vi "Loadcell CYL Home.vi"(7 "Model Name":T1, 8 "Error In":errorcluster, 9 "Intialize?":bool=TRUE, 10 "Inputs":T2) -> (0 "error out":errorcluster, 1 "Completed":bool, 4 "Status":cluster{"Status":string, "Elapsed Time":dbl})   [LabVIEW 2017]
uses:
  controls/All Inputs.ctl
  controls/SACB DI.ctl
  controls/Model Name.ctl
  controls/Loadcell CYL Home.ctl
  controls/FGV DO.ctl
panel:
  in  "Delay (for De-Clamp)":u32=500
  in  "Timeout (ms)":u32=15000
  # "Inputs"
  # "Variables"
  # "Outputs"
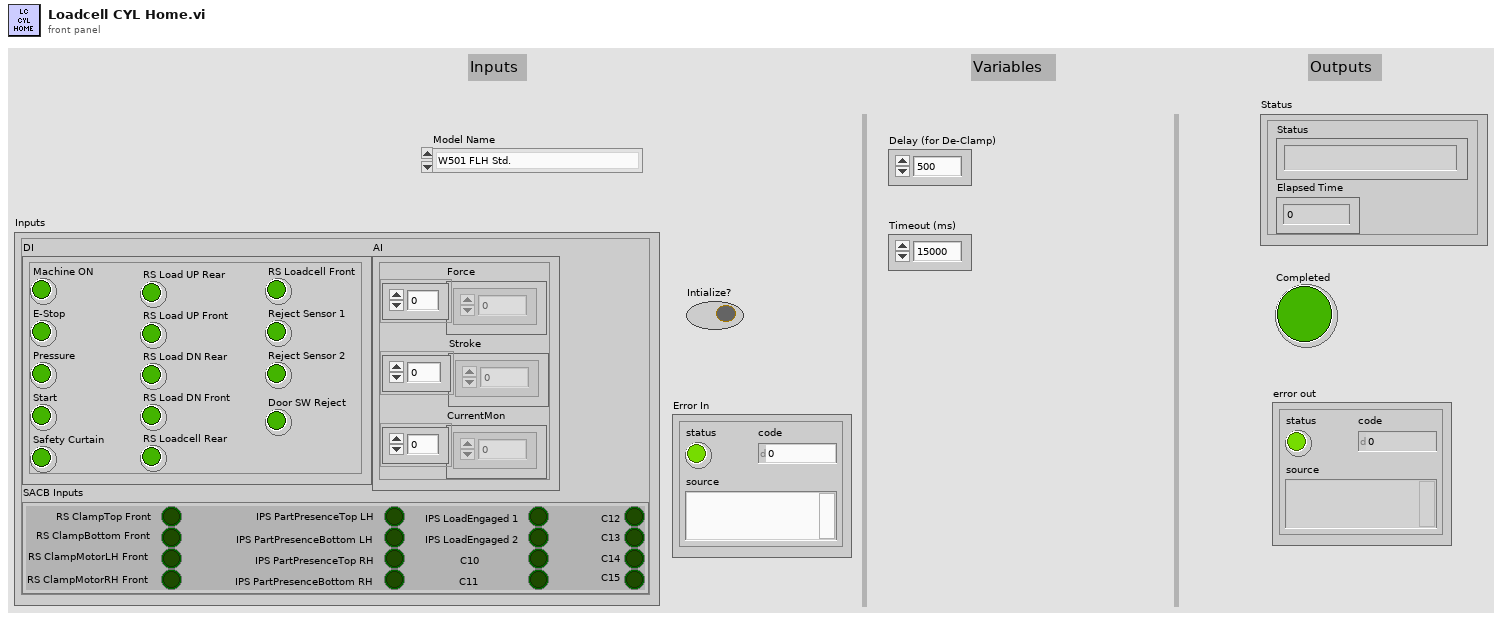
[diagram p1: front panel]
types:
  T1 = typedef "Model Name.ctl" = enum16{"W501 FLH Std.", "W501 FRH Std."}
  T2 = typedef "All Inputs.ctl" = cluster{"DI":cluster{"Machine ON":bool, "E-Stop":bool, "Pressure":bool, "Start":bool, "Safety Curtain":bool, "RS Load UP Rear":bool, "RS Load UP Front":bool, "RS Load DN Rear":bool, "RS Load DN Front":bool, "RS Loadcell Rear":bool, "RS Loadcell Front":bool, "Reject Sensor 1":bool, "Reject Sensor 2":bool, "Door SW Reject":bool}, "AI":cluster{"Force":dbl[], "Stroke":dbl[], "CurrentMon":dbl[]}, "SACB Inputs":T3}
  T3 = typedef "SACB DI.ctl" = cluster{"RS ClampTop Front":bool, "RS ClampBottom Front":bool, "RS ClampMotorLH Front":bool, "RS ClampMotorRH Front":bool, "IPS PartPresenceTop LH":bool, "IPS PartPresenceBottom LH":bool, "IPS PartPresenceTop RH":bool, "IPS PartPresenceBottom RH":bool, "IPS LoadEngaged 1":bool, "IPS LoadEngaged 2":bool, "C10":bool, "C11":bool, "C12":bool, "C13":bool, "C14":bool, "C15":bool}
  T4 = typedef "Loadcell CYL Home.ctl" = enum16{"Initialize", "Loadcell CYL to Home", "Delay", "Done", "Error"}
  T5 = typedef "FGV DO.ctl" = enum16{"Initialize", "Start Task", "Clamping", "Load CYL", "Contactors", "Loadcell CYL", "BSL", "Read DO", "Clear Tasks", "Clear Task"}
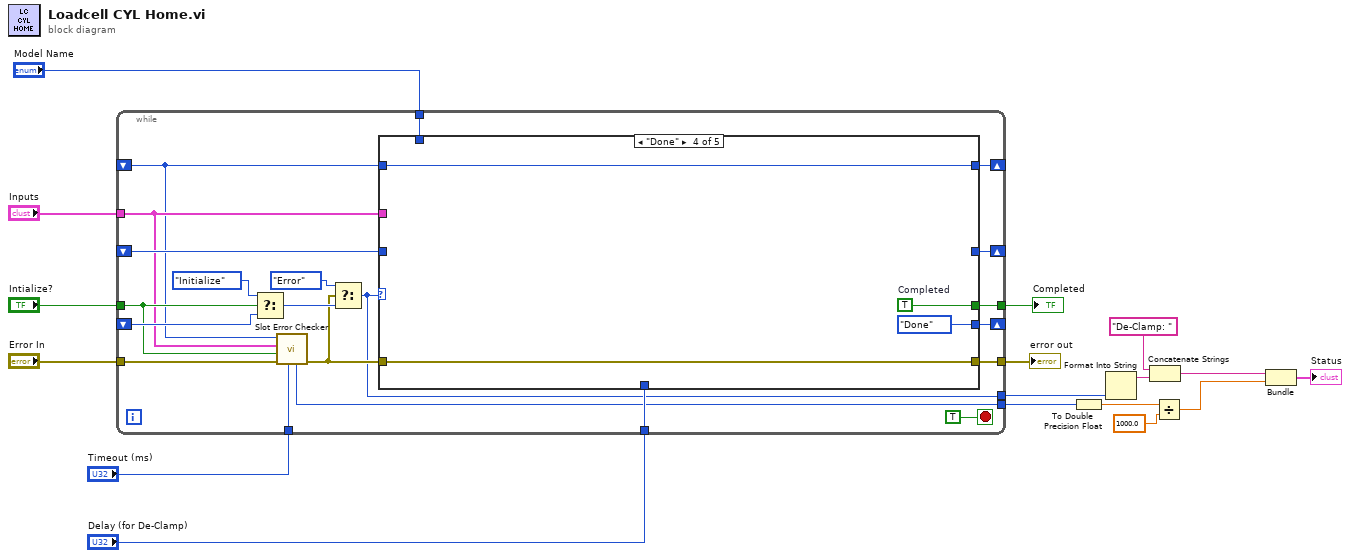
[diagram p0: block diagram]
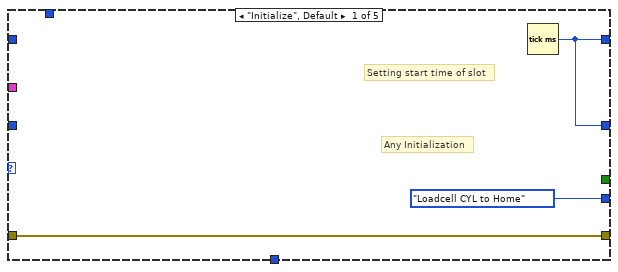
[diagram p2: hidden frame]
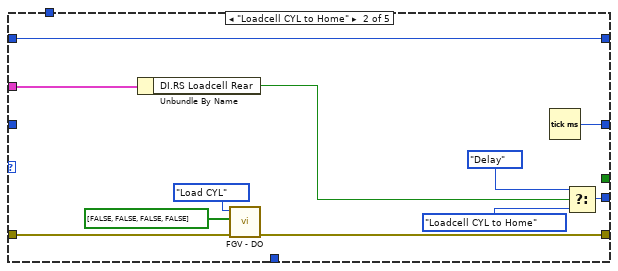
[diagram p3: hidden frame]
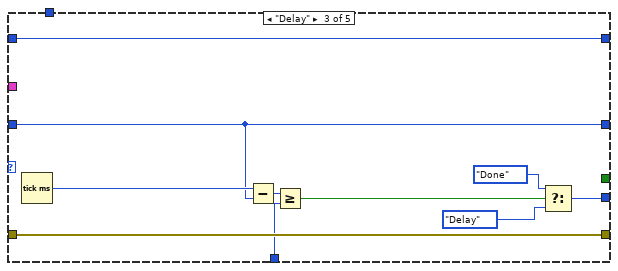
[diagram p4: hidden frame]
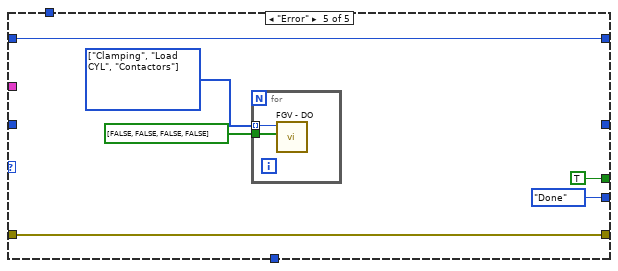
[diagram p5: hidden frame]
diagram:
  n1 = while {
    tunnel: "Intialize?" -> [w28]
    shift-right: [w35] -> _
    shift-left: _ -> [w37]
    shift-right: [w34] -> _
    shift-left: _ -> [w33]
    tunnel: "Error In" -> [w29]
    tunnel: [w32] -> w17
    tunnel: [w31] -> w16
    tunnel: "Inputs" -> [w27]
    shift-right: [w30] -> _
    shift-left: _ -> [w26]
    tunnel: "Delay (for De-Clamp)" -> [w22]
    tunnel: "Timeout (ms)" -> [w21]
    tunnel: [w20] -> w10
    tunnel: [w19] -> w7
    tunnel: "Model Name" -> [w18]
    stop <- TRUE stop-if-true
    n2 = Select(t=Loadcell_CYL_Home."Initialize", s=w28, f=w37) -> (s? t:f=w25:T4)
    n3 = call "Slot Error Checker.vi"("Timeout (ms)"=w21, "error in (no error)"=w29, "Intialize?"=w28, "Inputs"=w27, "start time"=w26) -> ("error out"=w24:errorcluster, "Slot Time"=w19:u32)  [unwired: 5 in]
    n4 = Select(t=Loadcell_CYL_Home."Error", s=w24, f=w25) -> (s? t:f=w20:T4)
    n5 = case shown="\"Done\"" w20 {
      tunnel: [Loadcell_CYL_Home."Loadcell CYL to Home" w45 w59 Loadcell_CYL_Home."Done" Loadcell_CYL_Home."Done"] -> w35
      tunnel: [w39 w48 w61 _ _] -> w34
      tunnel: w33 -> [_ _ w61 _ _]
      tunnel: w24 -> [w40 w52 w57 w65 w72]
      tunnel: [w40 w51 w57 w65 w72] -> w32
      tunnel: [_ _ _ w64 TRUE ("Completed")] -> w31
      tunnel: w27 -> [_ w46 _ _ _]
      tunnel: [w39 w47 w54 w63 w69] -> w30
      tunnel: w26 -> [_ w47 w54 w63 w69]
      tunnel: w22 -> [_ _ w53 _ _]
      tunnel: w18 -> [_ _ _ _ _]
      frame "Initialize", Default {
        # "Setting start time of slot"
        # "Any Initialization"
        n6 = Tick Count (ms)() -> (millisecond timer value=w39:u32)
      }
      frame "Loadcell CYL to Home" {
        n7 = Unbundle By Name(w46) -> ("DI.RS Loadcell Rear"=w42:bool)
        n8 = call "FGV - DO.vi"("error in"=w52, "Digital Outs"=bool[] [FALSE, FALSE, FALSE, FALSE], "State"=FGV_DO."Load CYL") -> ("error out"=w51:errorcluster)  [unwired: 7 in, 1 out]
        n9 = Tick Count (ms)() -> (millisecond timer value=w48:u32)
        n10 = Select(t=Loadcell_CYL_Home."Delay", s=w42, f=Loadcell_CYL_Home."Loadcell CYL to Home") -> (s? t:f=w45:T4)
      }
      frame "Delay" {
        n11 = Tick Count (ms)() -> (millisecond timer value=w62:u32)
        n12 = Subtract(x=w62, y=w61) -> (x-y=w60:u32)
        n13 = Greater Or Equal?(x=w60, y=w53) -> (x >= y?=w58:bool)
        n14 = Select(t=Loadcell_CYL_Home."Done", s=w58, f=Loadcell_CYL_Home."Delay") -> (s? t:f=w59:T4)
      }
      frame "Done" {
        w64 = TRUE  # Completed
      }
      frame "Error" {
        w67 = T5[] [enum."Clamping", enum."Load CYL", enum."Contactors"] items=["Initialize", "Start Task", "Clamping", "Load CYL", "Contactors", "Loadcell CYL", "BSL", "Read DO", "Clear Tasks", "Clear Task"]
        n15 = for {
          tunnel: w67 -> [w74] mode=indexing
          tunnel: bool[] [FALSE, FALSE, FALSE, FALSE] ("Digital Outs") -> [w73]
          n16 = call "FGV - DO.vi"("Digital Outs"=w73, "State"=w74) -> ()  [unwired: 8 in, 2 out]
        }
      }
    }
  }
  "error out" <- w17
  "Completed" <- w16
  n17 = To Double Precision Float(number=w7) -> (double precision float=w6:dbl)
  n18 = Format Into String(w10) -> (resulting string=w9:string)  [unwired: 3 in, 1 out]
  n19 = Concatenate Strings("De-Clamp: ", w9) -> (w4:string)
  n20 = Divide(x=w6, y=1000.0) -> (x/y=w3:dbl)
  n21 = Bundle(w4, w3) -> (→"Status":cluster{string, dbl})  [unwired: 1 in]
